vi "encode.vi"() -> ()   [LabVIEW 2018, in "posit.lvlib"]
uses:
  posit.lvlib
  unpacked.ctl
panel:
  in  "x":T1
  out "y":i16
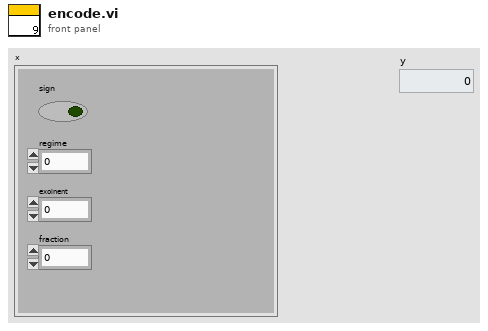
[diagram p1: front panel]
types:
  T1 = typedef "posit.lvlib/unpacked.ctl" = cluster{"sign":bool, "regime":i16, "exoinent":i16, "fraction":i16}
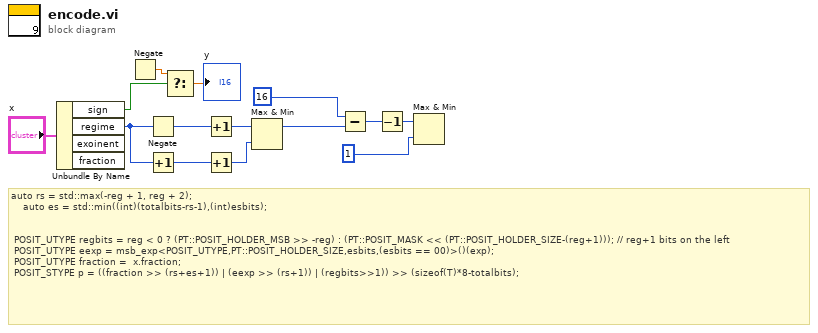
[diagram p0: block diagram]
diagram:
  # "auto rs = std::max(-reg + 1, reg + 2); \n    auto es = std::min((int)(totalbits-rs-1),(int)esbits);\n\n\n POSIT_UTYPE regbits = reg < 0 ? (PT::POSIT_HOLDER_MSB >> -reg) : (PT::POSIT_MASK << (PT::POSIT_HOLDER_SIZE-(reg+1))); // reg+1 bits on the left\n\tPOSIT_UTYPE eexp = msb_exp<POSIT_UTYPE,PT::POSIT_HOLDER_SIZE,esbits,(esbits == 00)>()(exp);\n\tPOSIT_UTYPE fraction =  x.fraction;\n\tPOSIT_STYPE p = ((fraction >> (rs+es+1)) | (eexp >> (rs+1)) | (regbits>>1)) >> (sizeof(T)*8-totalbits);"
  n1 = Unbundle By Name("x") -> ("sign"=w13:bool, "regime"=w7:i16)  [unwired: 2 out]
  n2 = Negate() -> (-x=w12:dbl)  [unwired: 1 in]
  n3 = Negate(x=w7) -> (-x=w10:i16)
  n4 = Increment(x=w7) -> (x+1=w8:i16)
  n5 = Select(t=w12, s=w13) -> (s? t:f=→"y":dbl)  [unwired: 1 in]
  n6 = Increment(x=w10) -> (x+1=w9:i16)
  n7 = Increment(x=w8) -> (x+1=w6:i16)
  n8 = Max & Min(x=w9, y=w6) -> (max(x,y)=w2:i16)  [unwired: 1 out]
  n9 = Subtract(x=i16 16, y=w2) -> (x-y=w5:i16)
  n10 = Decrement(x=w5) -> (x-1=w4:i16)
  n11 = Max & Min(x=w4, y=i16 1) -> ()  [unwired: 2 out]
